vi "CMD_LOADSTAMP.vi"(6 "Gantry in":refnum<class "Gantry.lvclass">, 8 "error in (no error)":errorcluster, 9 "Command":T1, 10 "Arguments":string[](array[string]), 11 "gScript Interpreter in":refnum<class "gScript Interpreter.lvclass">) -> (0 "error out":errorcluster, 3 "gScript Interpreter out":refnum<class "gScript Interpreter.lvclass">, 4 "Gantry out":refnum<class "Gantry.lvclass">)   [LabVIEW 2017, in "gScript Interpreter.lvclass"]
uses:
  gScript Interpreter.lvclass
  Shared Components/Gantry Class/Gantry.lvclass
  Type Definitions/Command.ctl
  Shared Components/FlexWorktable/FlexWorktable.lvclass
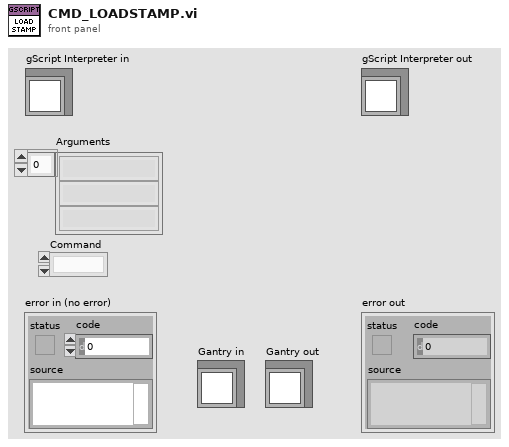
[diagram p1: front panel]
types:
  T1 = typedef "Command.ctl" = enum16{"", "PASS", "COPY", "PRINT", "GOTO", "GOTOIF", "GOTOIFN", "ADD", "SUB", "INC", "DEC", "HOME", "MOVEREL", "MOVENAME", "MOVETO", "GETPOS", "ROTATE", "GETROT", "SETVAC", "GETVAC", "JOYSTICK", "LOADTOOL", "UNLOADTOOL", "POTLINE", "POTDOT", "AUTOFOCUS", "FINDFID", "FIT", "WAIT", "MPGON", "MPGOFF", "PAUSE", "SNAPSHOT", "SETLOG", "CLEARLOG", "VIDEO", "TRANSFORMG2L", "TRANSFORML2G", "CHOICEPOPUP", "SETLIGHT", "CALL", "END", "DUMPSTATE", "FLEXREAD", "FLEXWRITE", "SURVEY", "LOADCONFIG", "SETERRORMODE", "COMPOSE", "INVERT", "EULER2QUAT", "QUAT2EULER", "MUL", "ROTATETO", "VERSION", "SIN", "COS", "TAN", "ATAN2", "ABS", "POW", "ACKFAULT", "MOVESAFE", "LOADSTAMP", "APPLYSTAMP", "UNLOADSTAMP", "LOADWEIGHT", "APPLYWEIGHT", "UNLOADWEIGHT"}
  T2 = typedef "Memory Cell.ctl" = cluster{"type":T3, "x":dbl, "y":dbl, "z":dbl, "w":dbl}
  T3 = typedef "Memory Cell Type Enum.ctl" = enum16{"integer", "float", "vector", "rotation"}
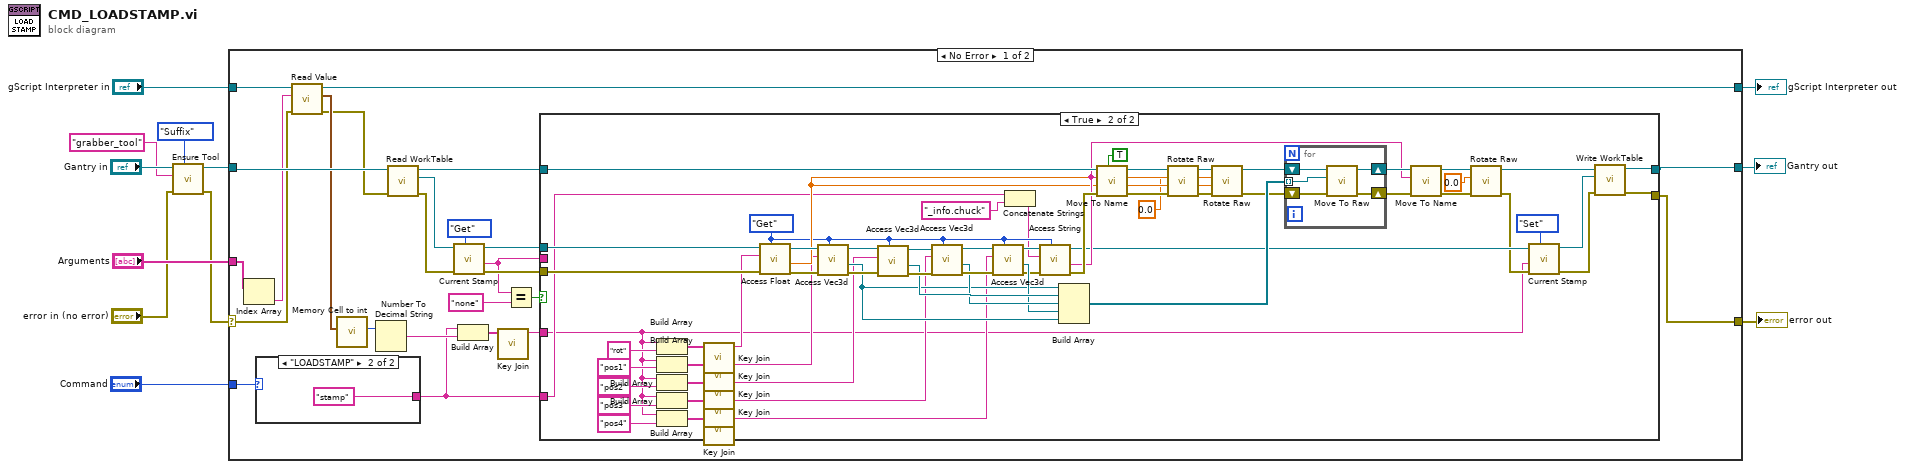
[diagram p0: block diagram]
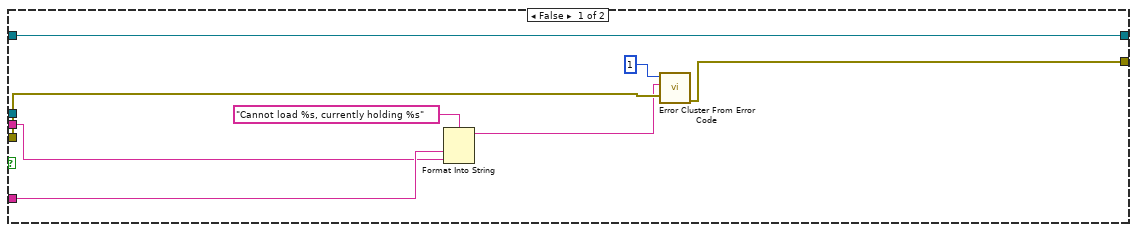
[diagram p2: hidden frame]
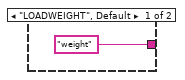
[diagram p3: hidden frame]
diagram:
  n1 = call "Ensure Tool.vi"("Match Type"=enum16{"Full", "Suffix"}."Suffix", "error in (no error)"="error in (no error)", "Tool Name"="grabber_tool", "Gantry in"="Gantry in") -> ("error out"=w3:errorcluster, "Gantry out"=w6:refnum<class "Gantry.lvclass">)  [unwired: 6 in]
  n2 = case shown="No Error" w3 {
    selector: w3 -> [w25 w117]
    tunnel: [w13 w117] -> w12
    tunnel: [w27 w116] -> w10
    tunnel: "gScript Interpreter in" -> [w28 w116]
    tunnel: "Arguments" -> [w37 _]
    tunnel: w6 -> [w36 w115]
    tunnel: [w19 w115] -> w8
    tunnel: "Command" -> [w21 _]
    frame No Error {
      n3 = Index Array(array=w37) -> (element=w26:string)  [unwired: 1 in]
      n4 = case shown="\"LOADSTAMP\"" w21 {
        tunnel: ["weight" "stamp"] -> w16
        frame "LOADWEIGHT", Default {
        }
        frame "LOADSTAMP" {
        }
      }
      n5 = call-dynamic "Read Value.vi"("error in (no error)"=w25, "String in"=w26, "gScript Interpreter in"=w28) -> ("error out"=w23:errorcluster, "Memory Cell"=w24:T2, "gScript Interpreter out"=w27:refnum<class "gScript Interpreter.lvclass">)  [unwired: 6 in]
      n6 = call "Memory Cell to int.vi"("Memory Cell"=w24) -> ("Int out"=w22:i32)  [unwired: 10 in]
      n7 = Number To Decimal String(number=w22) -> (decimal integer string=w17:string)  [unwired: 1 in]
      n8 = call-dynamic "Read WorkTable.vi"("error in"=w23, "Gantry Class in"=w36) -> ("error out"=w35:errorcluster, "Worktable"=w34:refnum<class "FlexWorktable.lvclass">, "Gantry Class out"=w30:refnum<class "Gantry.lvclass">)  [unwired: 7 in]
      n9 = call "Current Stamp.vi"("Get/Set"=enum16{"Get", "Set"}."Get", "error in (no error)"=w35, "FlexWorktable in"=w34) -> ("error out"=w31:errorcluster, "Current Stamp"=w18:string, "FlexWorktable out"=w29:refnum<class "FlexWorktable.lvclass">)  [unwired: 6 in]
      n10 = Build Array(w16, w17) -> (w15:string[])
      n11 = call "Key Join.vi"("Key Elements"=w15) -> ("Key"=w14:string)  [unwired: 10 in]
      n12 = Equal?(x=w18, y="none") -> (x = y?=w32:bool)
      n13 = case shown="True" w32 {
        tunnel: [w43 w48] -> w13
        tunnel: w31 -> [w44 w93]
        tunnel: w30 -> [w42 w90]
        tunnel: [w42 w49] -> w19
        tunnel: w29 -> [_ w105]
        tunnel: w16 -> [_ w55]
        tunnel: w18 -> [w38 _]
        tunnel: w14 -> [w39 w46]
        frame False {
          n14 = Format Into String(format string="Cannot load %s, currently holding %s" ("error message (\"\")"), w39, w38) -> (resulting string=w40:string)  [unwired: 2 in, 1 out]
          n15 = call <vilib>:"Error Cluster From Error Code.vi"("error in (no error)"=w44, "error message (\"\")"=w40, "error code (0)"=1) -> ("error out"=w43:errorcluster)  [unwired: 6 in]
        }
        frame True {
          w73 = enum16{"Get", "Set"}."Get" ("Get/Set")
          n16 = Build Array(w46, "rot" ("string")) -> (w67:string[])
          n17 = Build Array(w46, "pos1" ("string")) -> (w65:string[])
          n18 = Build Array(w46, "pos2" ("string")) -> (w64:string[])
          n19 = Build Array(w46, "pos3" ("string")) -> (w63:string[])
          n20 = Build Array(w46, "pos4" ("string")) -> (w66:string[])
          n21 = call "Key Join.vi"("Key Elements"=w67) -> ("Key"=w62:string)  [unwired: 10 in]
          n22 = call "Key Join.vi"("Key Elements"=w65) -> ("Key"=w61:string)  [unwired: 10 in]
          n23 = call "Key Join.vi"("Key Elements"=w64) -> ("Key"=w60:string)  [unwired: 10 in]
          n24 = call "Key Join.vi"("Key Elements"=w63) -> ("Key"=w59:string)  [unwired: 10 in]
          n25 = call "Key Join.vi"("Key Elements"=w66) -> ("Key"=w58:string)  [unwired: 10 in]
          n26 = call-dynamic "Access Float.vi"("Get/Set"=w73, "error in (no error)"=w93, "Key"=w62, "FlexWorktable in"=w105) -> ("error out"=w107:errorcluster, "Value out"=w80:dbl, "FlexWorktable out"=w106:refnum<class "FlexWorktable.lvclass">)  [unwired: 5 in]
          n27 = call-dynamic "Access Vec3d.vi"("Get/Set"=w73, "error in (no error)"=w107, "Key"=w61, "FlexWorktable in"=w106) -> ("error out"=w104:errorcluster, "Value out"=w91:refnum<class "Vec3d.lvclass">, "FlexWorktable out"=w103:refnum<class "FlexWorktable.lvclass">)  [unwired: 5 in]
          n28 = call-dynamic "Access Vec3d.vi"("Get/Set"=w73, "error in (no error)"=w104, "Key"=w60, "FlexWorktable in"=w103) -> ("error out"=w102:errorcluster, "Value out"=w98:refnum<class "Vec3d.lvclass">, "FlexWorktable out"=w101:refnum<class "FlexWorktable.lvclass">)  [unwired: 5 in]
          n29 = call-dynamic "Access Vec3d.vi"("Get/Set"=w73, "error in (no error)"=w102, "Key"=w59, "FlexWorktable in"=w101) -> ("error out"=w100:errorcluster, "Value out"=w97:refnum<class "Vec3d.lvclass">, "FlexWorktable out"=w99:refnum<class "FlexWorktable.lvclass">)  [unwired: 5 in]
          n30 = call-dynamic "Access Vec3d.vi"("Get/Set"=w73, "error in (no error)"=w100, "Key"=w58, "FlexWorktable in"=w99) -> ("error out"=w87:errorcluster, "Value out"=w96:refnum<class "Vec3d.lvclass">, "FlexWorktable out"=w88:refnum<class "FlexWorktable.lvclass">)  [unwired: 5 in]
          n31 = Concatenate Strings(w55, "_info.chuck" ("Key")) -> (w57:string)
          n32 = call-dynamic "Access String.vi"("Get/Set"=w73, "error in (no error)"=w87, "Key"=w57, "FlexWorktable in"=w88) -> ("error out"=w89:errorcluster, "Value out"=w84:string, "FlexWorktable out"=w51:refnum<class "FlexWorktable.lvclass">)  [unwired: 5 in]
          n33 = Build Array(w91, w98, w97, w96, w91) -> (w95:refnum<class "Vec3d.lvclass">[])
          n34 = call-dynamic "Move To Name.vi"("Move if Same"=TRUE, "error in"=w89, "Destination"=w84, "Gantry in"=w90) -> ("error out"=w75:errorcluster, "Gantry out"=w78:refnum<class "Gantry.lvclass">)  [unwired: 6 in]
          n35 = call-dynamic "Rotate Raw.vi"("error in"=w75, "position(deg)"=0.0, "Gantry in"=w78) -> ("error out"=w76:errorcluster, "Gantry out"=w77:refnum<class "Gantry.lvclass">)  [unwired: 7 in]
          n36 = call-dynamic "Rotate Raw.vi"("error in"=w76, "speed(deg/s)"=w80, "position(deg)"=w80, "Gantry in"=w77) -> ("error out"=w92:errorcluster, "Gantry out"=w94:refnum<class "Gantry.lvclass">)  [unwired: 6 in]
          n37 = for {
            tunnel: w95 -> [w112] mode=indexing
            shift-right: [w109] -> w85
            shift-left: w92 -> [w108]
            shift-right: [w110] -> w86
            shift-left: w94 -> [w111]
            n38 = call-dynamic "Move To Raw.vi"("error in"=w108, "Destination"=w112, "Gantry in"=w111) -> ("error out"=w109:errorcluster, "Gantry out"=w110:refnum<class "Gantry.lvclass">)  [unwired: 7 in]
          }
          n39 = call-dynamic "Move To Name.vi"("error in"=w85, "Destination"=w84, "Gantry in"=w86) -> ("error out"=w81:errorcluster, "Gantry out"=w82:refnum<class "Gantry.lvclass">)  [unwired: 7 in]
          n40 = call-dynamic "Rotate Raw.vi"("error in"=w81, "position(deg)"=0.0, "Gantry in"=w82) -> ("error out"=w47:errorcluster, "Gantry out"=w50:refnum<class "Gantry.lvclass">)  [unwired: 7 in]
          n41 = call "Current Stamp.vi"("Get/Set"=enum16{"Get", "Set"}."Set", "error in (no error)"=w47, "New Stamp"=w46, "FlexWorktable in"=w51) -> ("error out"=w54:errorcluster, "FlexWorktable out"=w53:refnum<class "FlexWorktable.lvclass">)  [unwired: 5 in, 1 out]
          n42 = call-dynamic "Write WorkTable.vi"("error in (no error)"=w54, "FlexWorktable"=w53, "Gantry Class in"=w50) -> ("error out"=w48:errorcluster, "Gantry Class out"=w49:refnum<class "Gantry.lvclass">)  [unwired: 7 in]
        }
      }
    }
    frame Error {
    }
  }
  "error out" <- w12
  "gScript Interpreter out" <- w10
  "Gantry out" <- w8
